vi "Q14070-Z120主界面111.vi"() -> ()   [LabVIEW 2013]
uses:
  <vilib>/printing/EasyPrintingControls.llb/contents.ctl
  <vilib>/printing/EasyPrintingControls.llb/report_type.ctl
  <vilib>/Utility/NIReport.llb/NI_report.lvclass
  <vilib>/printing/EasyPrinting.llb/Easy Print VI Panel or Documentation (path).vi
  PCI8622_32.dll
  <vilib>/Utility/NIReport.llb/NI_ReportGenerationCore.lvlib
panel:
  out "伺服慢进速度":dbl
  out "右伺服慢进位置":dbl format="%#.2f"
  out "左伺服慢进位置":dbl format="%#.2f"
  out "JSSJ":string
  out "FGCS":string
  out "KSSJ":string
  out "本序合格":bool
  out "右压力参数组":dbl[](array[numeric])
  out "右位移参数组":dbl[](array[numeric])
  out "左压力参数组":dbl[](array[numeric])
  out "左位移参数组":dbl[](array[numeric])
  out "右伺服设定走位":dbl
  out "左伺服设定走位":dbl
  out "程序选择-2":bool
  out "程序选择-1":bool
  out "工步提示2":string
  out "工步提示1":string
  in  "报警工步号":u32 caption="工步号1"
  out "报警提示":string
  in  "自动工步号":u32 caption="工步号1"
  out "自动工步提示":string
  in  "产品ID":string="201209190001"
  in  "员工ID":string
  out "员工姓名":string
  in  "电动缸全回零":bool
  in  "电动缸全复位":bool
  out "右伺服快进位置":dbl format="%#.2f"
  out "左伺服快进位置":dbl format="%#.2f"
  out "伺服快进速度":dbl
  out "参数保存错误":errorcluster
  out "传感器保存错误":errorcluster
  out "左实时压力(N)":dbl format="%#.3f"
  out "左实时位移(mm)":dbl=10000.0 format="%#.2f"
  out "右实时位移(mm)":dbl=10000.0 format="%#.2f"
  out "右实时压力(N)":dbl format="%#.3f"
  out "右压装合格":bool
  out "右压装不合格":bool
  out "左压装不合格":bool
  out "左压装合格":bool
  out "监控点最大压力2(KN)":dbl format="%#.3f"
  out "监控点最小压力2(KN)":dbl format="%#.3f"
  out "区域最小压力2(KN)":dbl format="%#.3f"
  out "区域最大压力2(KN)":dbl format="%#.3f"
  out "区域最小位移2(mm)":dbl format="%#.1f"
  out "区域最大位移2(mm)":dbl format="%#.1f"
  out "区域最小压力1(KN)":dbl format="%#.3f"
  out "监控点最大压力1(KN)":dbl format="%#.3f"
  out "监控点最小压力1(KN)":dbl format="%#.3f"
  out "区域最大压力1(KN)":dbl format="%#.3f"
  out "区域最小位移1(mm)":dbl format="%#.1f"
  out "区域最大位移1(mm)":dbl format="%#.1f"
  in  "左工步号2900":u32 caption="工步号1"
  in  "右工步号2700":u32 caption="工步号"
  in  "报警清除":bool
  in  "参数加载":bool
  in  "型号选择":u32(ring) items=["J706", "J709"]
  out "参数加载错误":errorcluster
  in  "停止":bool
  out "ADODB._Connection Out":refnum<k7>
  out "参数查询错误":errorcluster
  in  "联线按钮":bool
  out "通讯状态":bool
  in  "选项卡控件":T1(tab)
  out "左压力位移曲线":cluster{"Y":dbl[], "Y":dbl[]}[](graph) caption="XY图"
  out "右压力位移曲线":cluster{"Y":dbl[], "Y":dbl[]}[](graph) caption="XY图"
  out "压力报警1":bool
  out "压力报警2":bool
  out "左实测监控点压力1(KN)":dbl format="%#.3f"
  out "左实测压入位移(mm)":dbl format="%#.1f"
  out "左实测监控点压力2(KN)":dbl format="%#.3f"
  out "右实测监控点压力2(KN)":dbl format="%#.3f"
  out "右实测压入位移(mm)":dbl format="%#.1f"
  out "右实测监控点压力1(KN)":dbl format="%#.3f"
  out "位移监控点1(mm)":dbl format="%#.2f"
  out "位移监控点2(mm)":dbl format="%#.2f"
  out "右电动缸零位":bool
  out "左电动缸下限":bool
  out "右气缸下降":bool
  out "右气缸上升":bool
  out "右气缸下位":bool
  out "右气缸上位":bool
  out "左气缸上升":bool
  out "左气缸下降":bool
  out "左气缸上位":bool
  out "左气缸下位":bool
  out "左电动缸零位":bool
  out "右电动缸上限":bool
  out "右电动缸下限":bool
  out "左电动缸上限":bool
  in  "顶升气缸上升-右":bool
  in  "顶升气缸下降-右":bool
  in  "顶升气缸上升-左":bool
  in  "顶升气缸下降-左":bool
  out "启动2按钮":bool
  out "启动1按钮":bool
  out "手动/自动":bool
  out "复位按钮":bool
  in  "电动缸下降-右":bool
  in  "电动缸上升-右":bool
  in  "电动缸下降-左":bool
  in  "电动缸上升-左":bool
  in  "电动缸回零-右":bool
  in  "电动缸回零-左":bool
  in  "电动缸复位-左":bool
  in  "电动缸复位-右":bool
  out "急停按钮":bool
  out "安全光幕":bool
  out "气压报警":bool
  in  "右伺服设定走位":dbl caption="右伺服设定走位负值"
  in  "左伺服设定走位":dbl caption="左伺服设定走位负值"
  in  "电动缸绝对移动调试-右":bool
  in  "电动缸绝对移动调试-左":bool
  out "左伺服实时位置":dbl
  out "右伺服实时位置":dbl
  in  "电动缸复位-右 2":bool
  in  "电动缸复位-左 2":bool
  in  "电动缸回零-左 2":bool
  in  "电动缸回零-右 2":bool
  in  "电动缸下降-右 2":bool
  in  "电动缸上升-右 2":bool
  in  "电动缸下降-左 2":bool
  in  "电动缸上升-左 2":bool
  in  "传感器参数保存":bool
  in  "压力1零点偏移值":dbl format="%#.3f"
  in  "压力1比例偏移值":dbl format="%#.3f"
  in  "左位移比例偏移值":dbl format="%#.3f"
  in  "左位移零点偏移值":dbl format="%#.3f"
  in  "压力2零点偏移值":dbl format="%#.3f"
  in  "压力2比例偏移值":dbl format="%#.3f"
  in  "右位移比例偏移值":dbl format="%#.3f"
  in  "右位移零点偏移值":dbl format="%#.3f"
  in  "参数保存":bool
  in  "参数查询":bool
  in  "参数列表":string[][](table)
  # "Q14070-Z120压减震套"
  # "Copying (C) 2014 湖北唯思凌科装备制造有限公司 版权所有"
  # "此界面供伺服定位用，正常生产时 禁止操作！！！"
  # "传感器校验区"
  # "关于传感器校验：\n1、传感器校验需要由具备资质的单位或部门进行校验。\n2、具备权限的用户才能够修改传感器校验参数和试验参数。\n3、修改校验参数方法：先将比例偏移置为1，修改零点偏移，使零点值与校验的传感器一致；然后根据增幅调整比例偏移。"
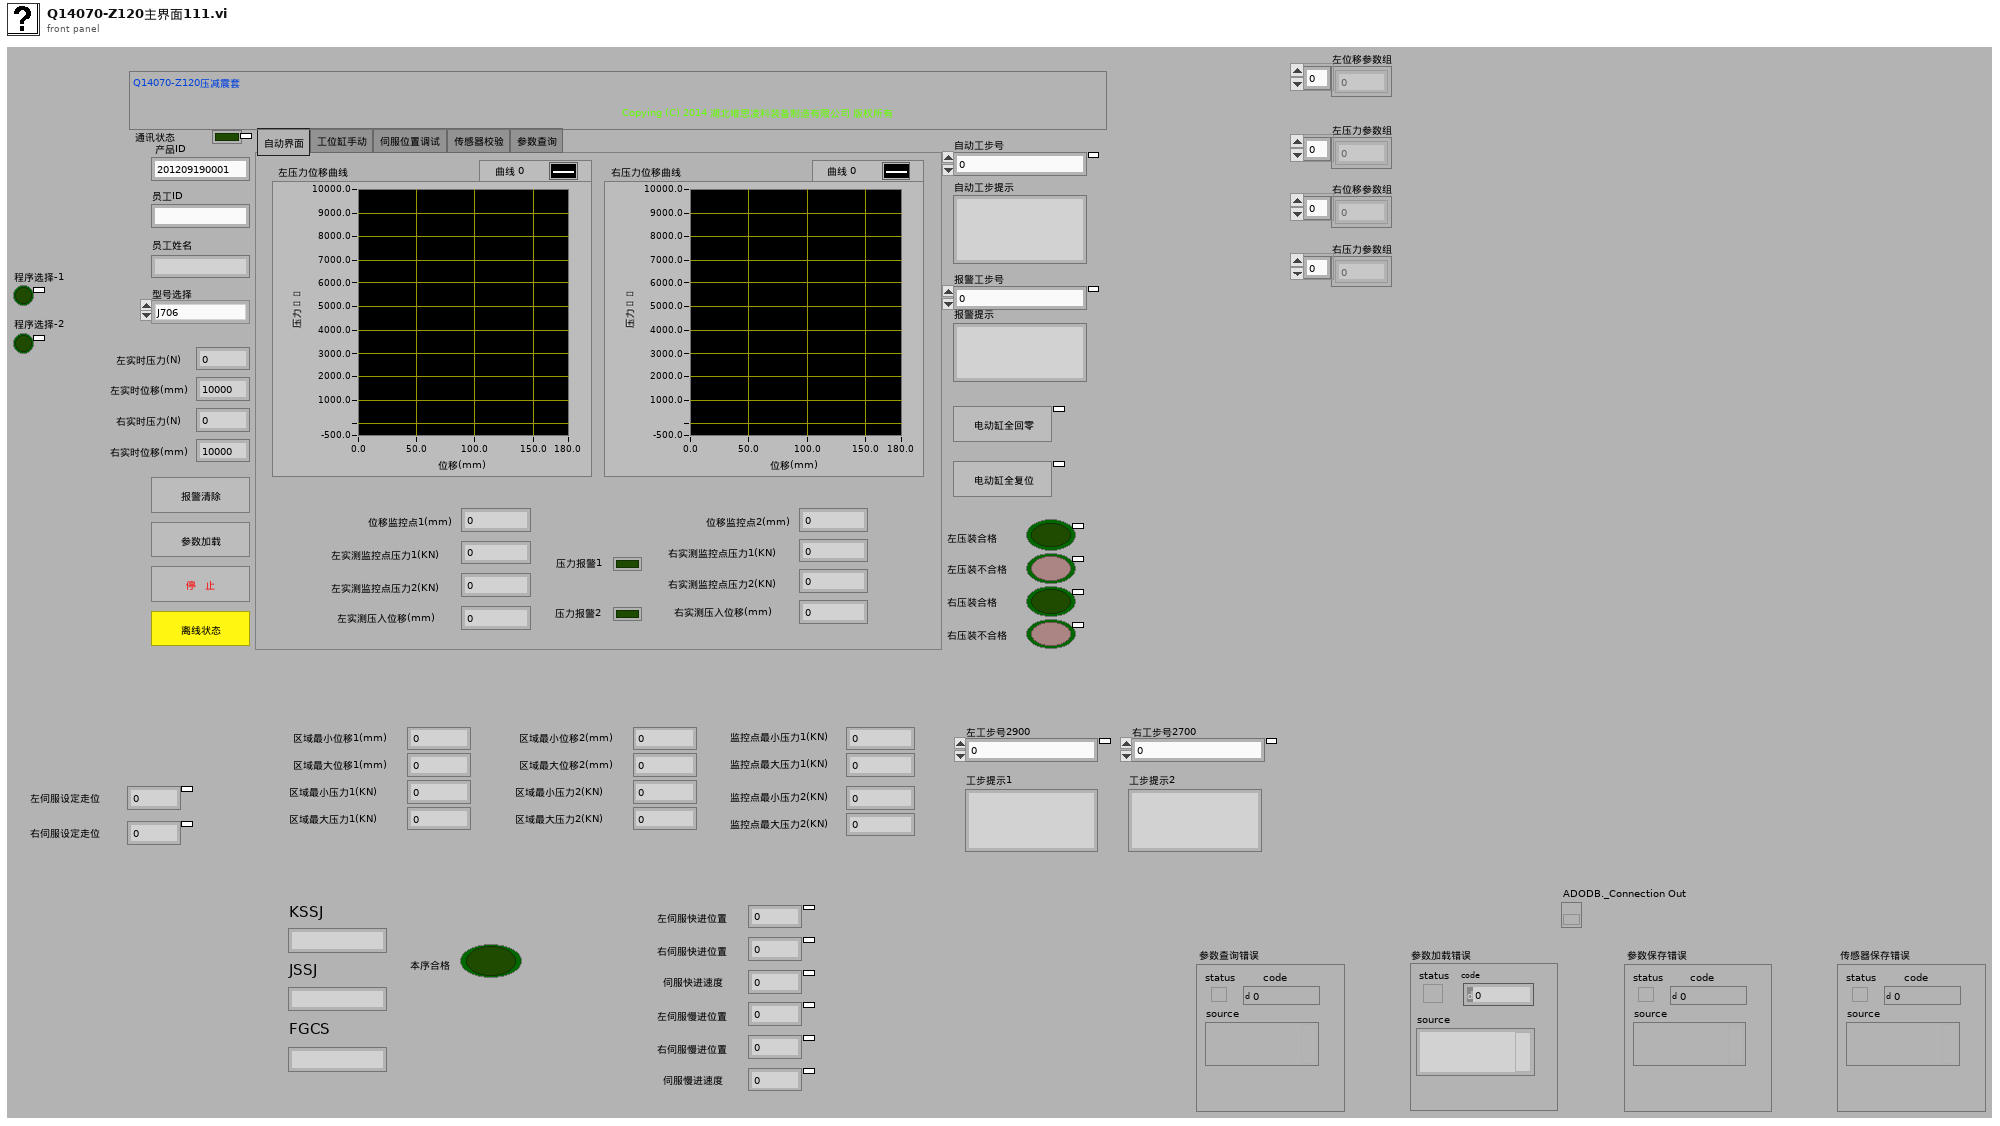
[diagram p1: front panel]
types:
  T1 = enum32{"自动界面", "工位缸手动", "伺服位置调试", "传感器校验", "参数查询"}
  T2 = enum32{"invalid app kind", "Development System", "Run Time System", "Student Edition", "Embedded LabVIEW", "Evaluation", "Custom"}
  T3 = typedef "NI_ReportGenerationCore.lvlib/report_type.ctl" = u16
  T4 = typedef "NI_ReportGenerationCore.lvlib/contents.ctl" = u16
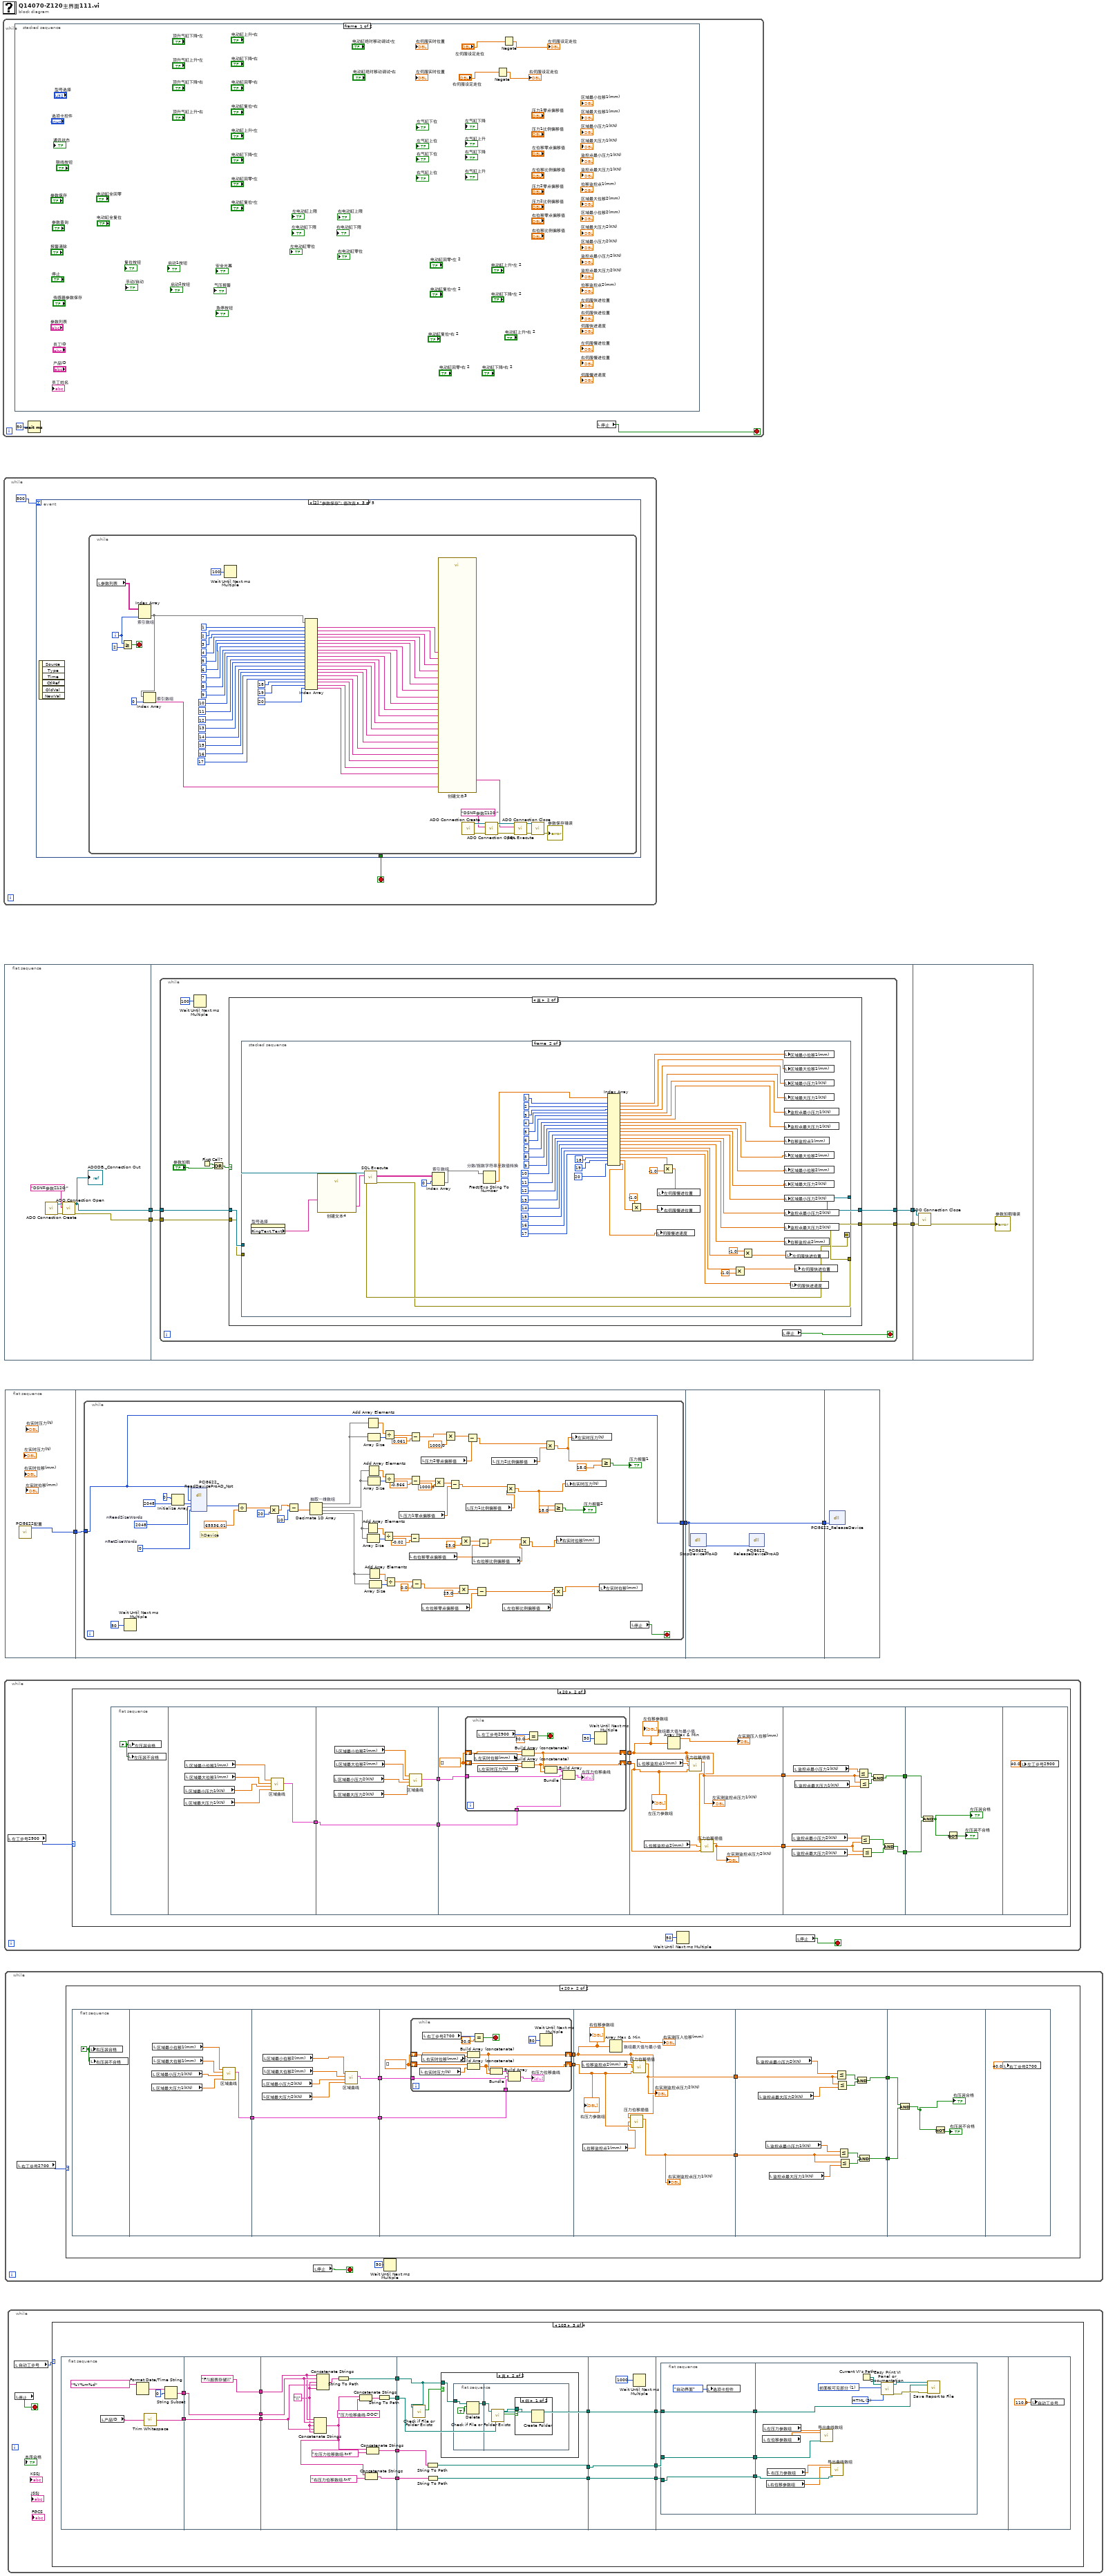
[diagram p0: block diagram]
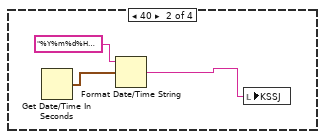
[diagram p3: hidden frame]
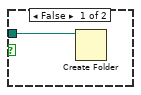
[diagram p4: hidden frame]
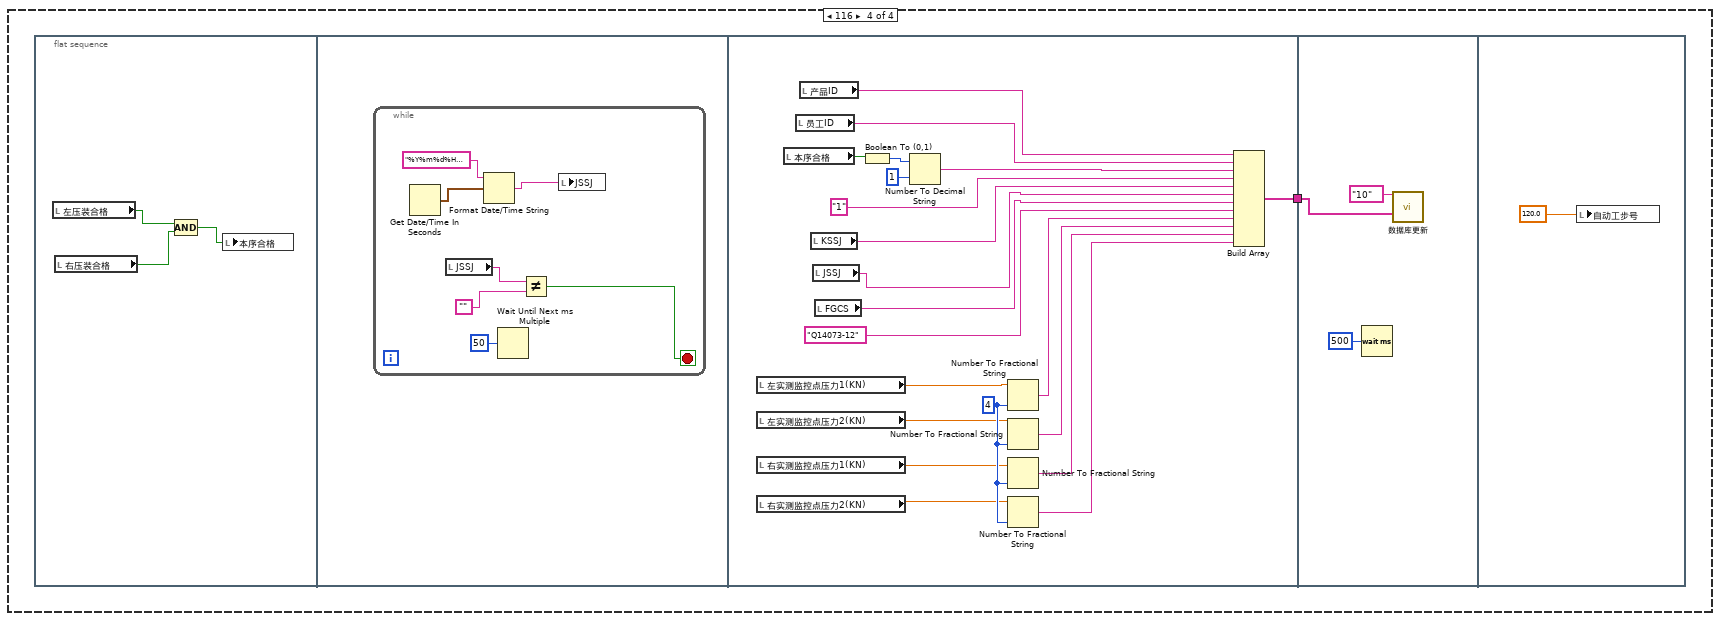
[diagram p6: hidden frame]
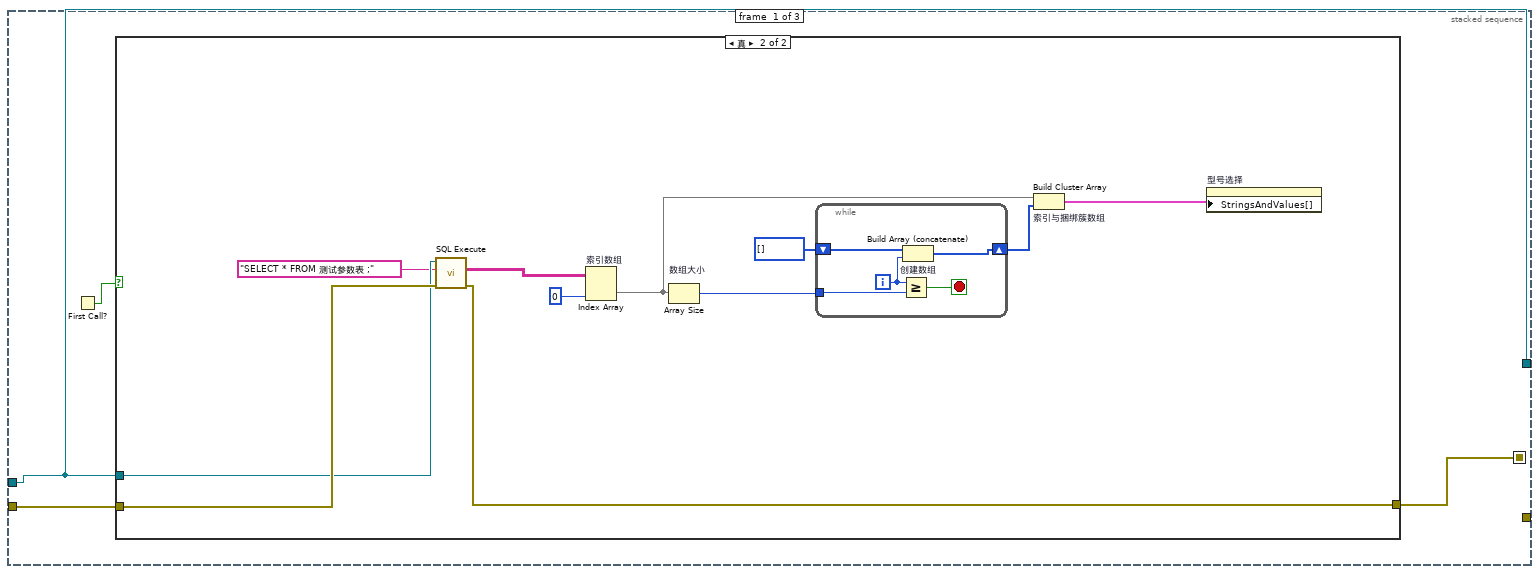
[diagram p10: hidden frame]
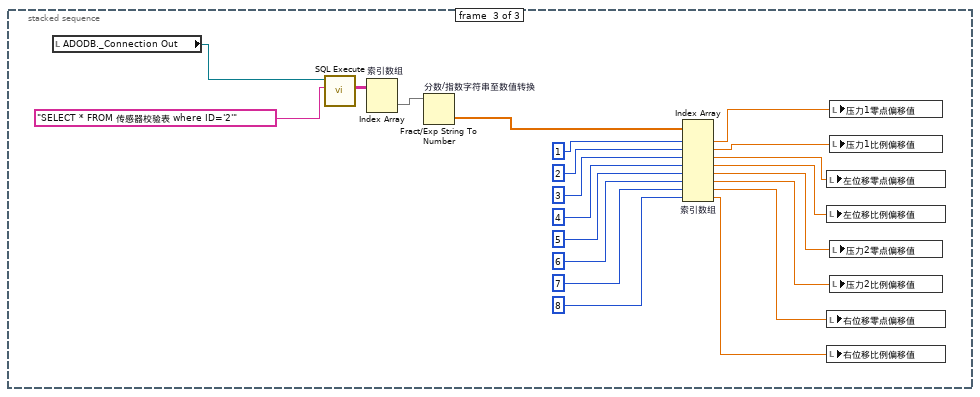
[diagram p12: hidden frame]
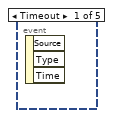
[diagram p13: hidden frame]
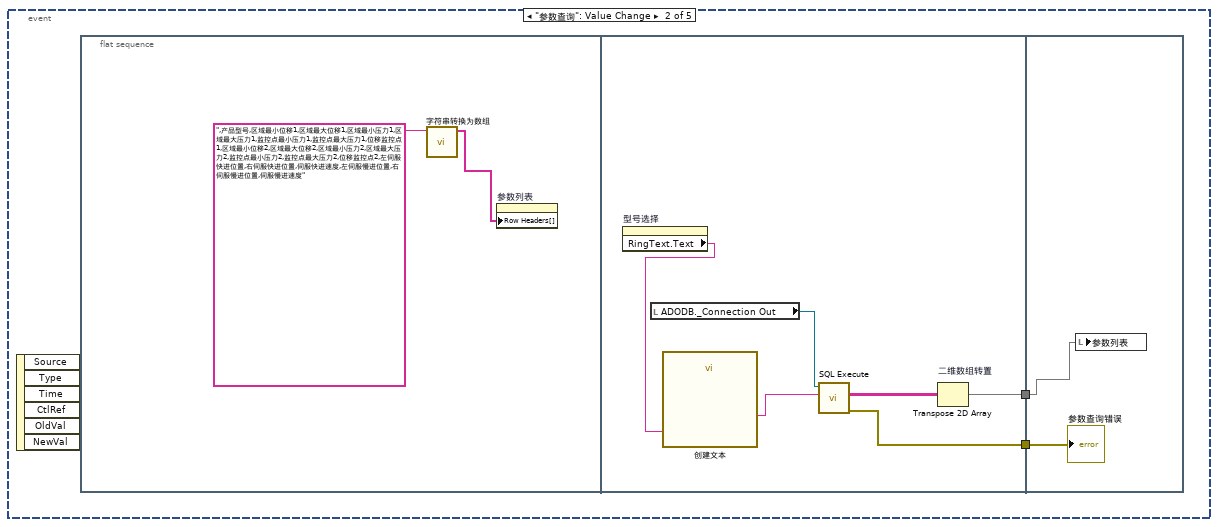
[diagram p14: hidden frame]
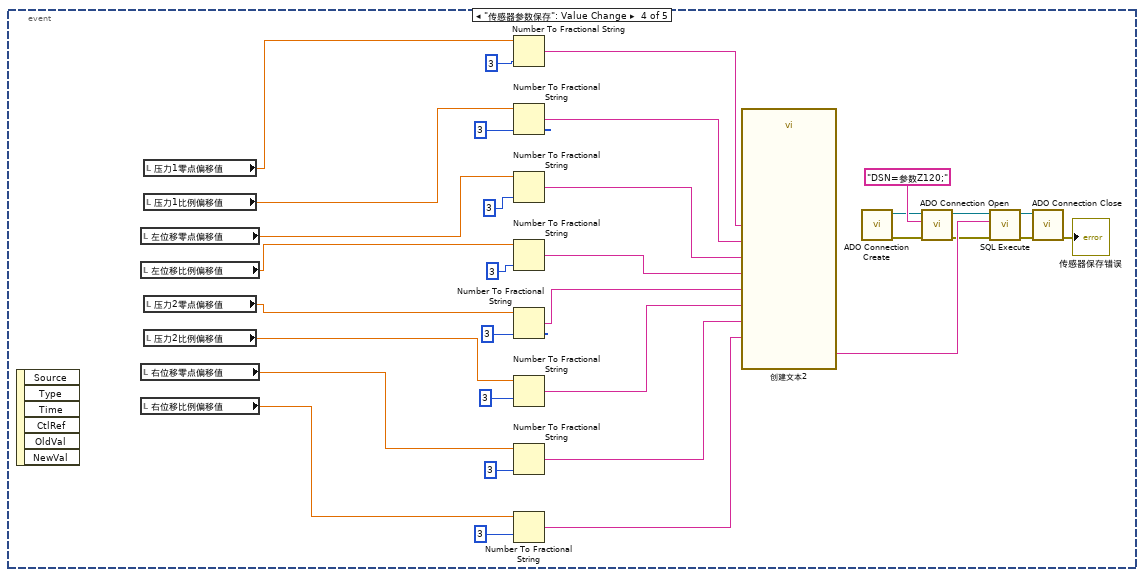
[diagram p15: hidden frame]
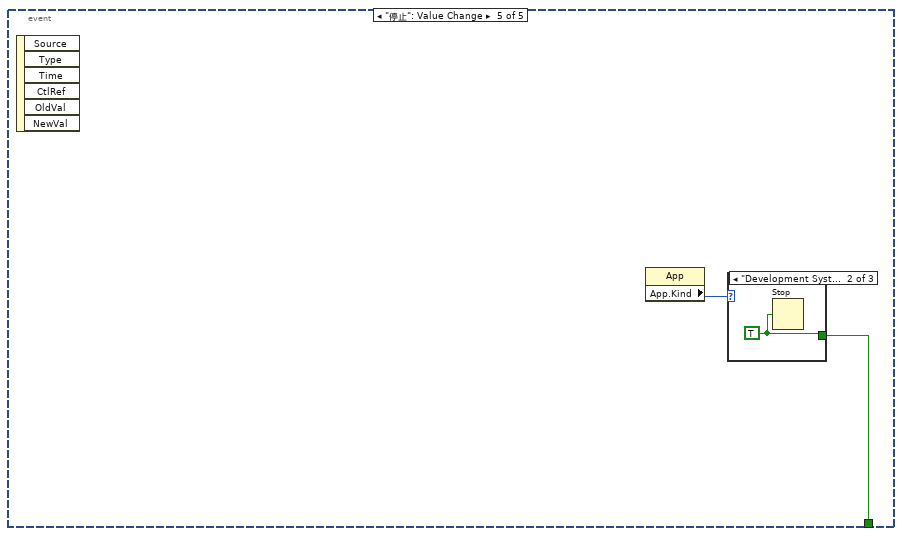
[diagram p16: hidden frame]
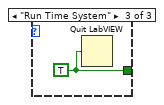
[diagram p18: hidden frame]
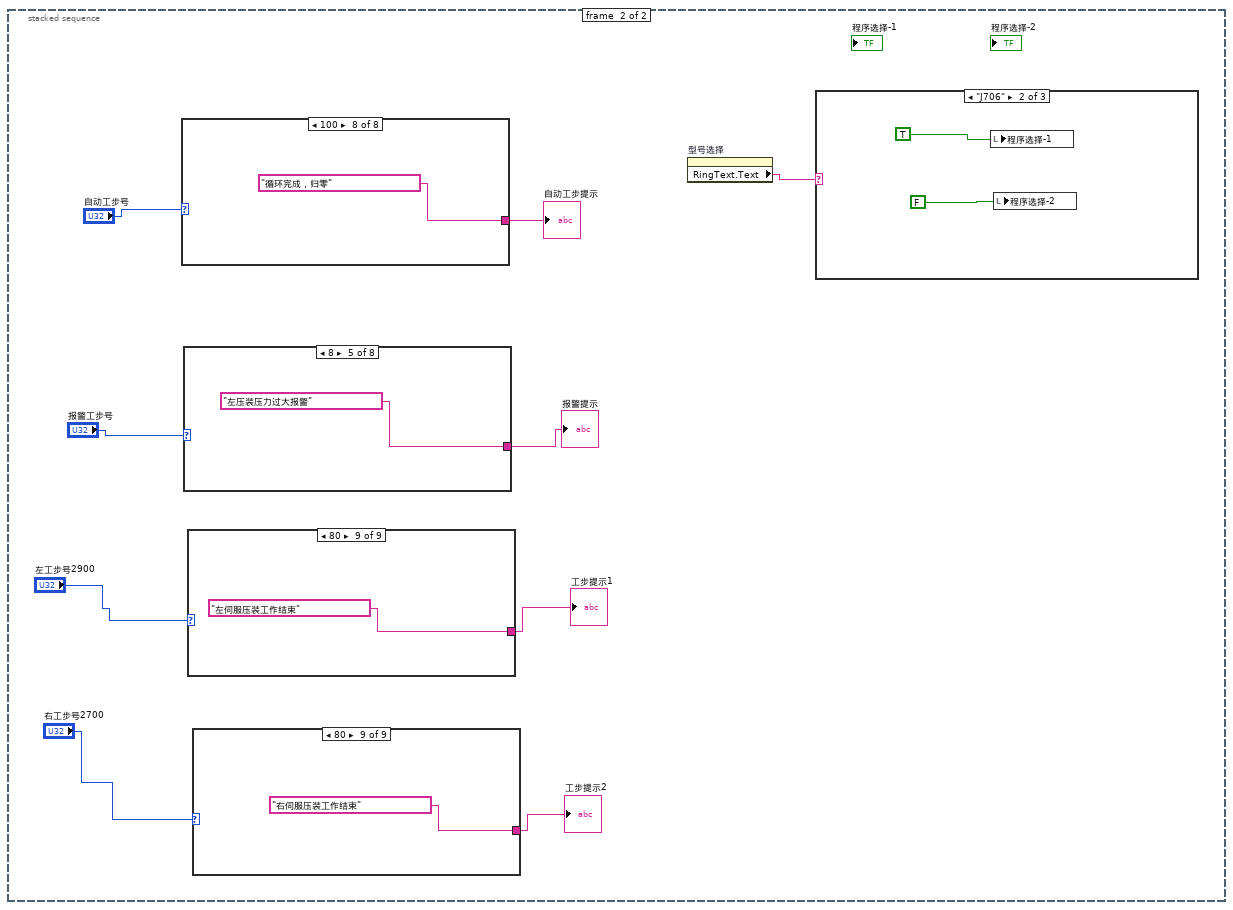
[diagram p19: hidden frame]
diagram:
  n1 = while {
    stop <- w8 stop-if-true
    n2 = stacked-sequence {
      frame #0 {
        n3 = Negate(x="右伺服设定走位") -> (-x=→"右伺服设定走位":dbl)
        n4 = Negate(x="左伺服设定走位") -> (-x=→"左伺服设定走位":dbl)
      }
      frame #1 {
        n5 = case shown="100" "自动工步号" {
          tunnel: ["放入工件，减震套，准备开始" "双手启动开始" "电动缸下降开始" "电动缸下降完成" "电动缸开始回零" "电动缸回零完成，顶升气缸顶升" "顶升气缸下降" "循环完成，归零"] -> w21
          frame 0, Default {
          }
          frame 40 {
          }
          frame 50 {
          }
          frame 60 {
          }
          frame 70 {
          }
          frame 80 {
          }
          frame 90 {
          }
          frame 100 {
          }
        }
        "自动工步提示" <- w21
        n6 = case shown="8" "报警工步号" {
          tunnel: ["工作正常" "压装过程触碰光幕，请急停后复位，并对电动缸回零" "左压装不合格" "右压装不合格" "左压装压力过大报警" "右压装压力过大报警" "左伺服报警，请复位伺服电机" "右伺服报警，请复位伺服电机"] -> w19
          frame 0, Default {
          }
          frame 2 {
          }
          frame 6 {
          }
          frame 7 {
          }
          frame 8 {
          }
          frame 9 {
          }
          frame 11 {
          }
          frame 12 {
          }
        }
        "报警提示" <- w19
        n7 = case shown="80" "左工步号2900" {
          tunnel: ["准备压装" "左伺服压装开始" "左伺服压装中" "左伺服压装结束" "左伺服曲线采集完成" "左伺服回零开始" "左伺服回零中" "左伺服回零完成" "左伺服压装工作结束"] -> w18
          frame 0, Default {
          }
          frame 10 {
          }
          frame 20 {
          }
          frame 30 {
          }
          frame 40 {
          }
          frame 50 {
          }
          frame 60 {
          }
          frame 70 {
          }
          frame 80 {
          }
        }
        "工步提示1" <- w18
        n8 = case shown="80" "右工步号2700" {
          tunnel: ["" "右伺服压装开始" "右伺服压装中" "右伺服压装结束" "右伺服曲线采集完成" "右伺服回零开始" "右伺服回零中" "右伺服回零完成" "右伺服压装工作结束"] -> w17
          frame 0, Default {
          }
          frame 10 {
          }
          frame 20 {
          }
          frame 30 {
          }
          frame 40 {
          }
          frame 50 {
          }
          frame 60 {
          }
          frame 70 {
          }
          frame 80 {
          }
        }
        "工步提示2" <- w17
        n9 = property on="型号选择" class="Ring (严格)"() -> ("RingText.Text"=w14:string)  [unwired: 2 in, 2 out]
        n10 = case shown="\"J706\"" w14 {
          frame "0", Default {
          }
          frame "J706" {
            n11 = local write "程序选择-1"(TRUE ("程序选择-1")) -> ()
            n12 = local write "程序选择-2"(FALSE ("程序选择-2")) -> ()
          }
          frame "J709" {
            n13 = local write "程序选择-1"(FALSE ("程序选择-1")) -> ()
            n14 = local write "程序选择-2"(TRUE ("程序选择-2")) -> ()
          }
        }
      }
    }
    n15 = Wait (ms)(milliseconds to wait=u32 50 ("毫秒倍数")) -> ()  [unwired: 1 out]
    n16 = local read "停止"() -> (w8:bool)
  }
  n17 = while {
    stop <- w61 stop-if-true
    n18 = event shown="[2] \"参数保存\": 值改变" {
      selector: _ -> [_ _ _ _ _]
      dyn-events: _ -> [_ _ _ _ _]
      timeout: 500 -> [_ _ _ _ _]
      tunnel: [_ _ _ _ w165] -> w61
      event Timeout {
        n19 = event-data() -> ()  [unwired: 1 in, 3 out]
      }
      event "参数查询": Value Change {
        n20 = event-data() -> ()  [unwired: 1 in, 6 out]
        n21 = flat-sequence {
          tunnel: [w70] -> w64
          tunnel: [w69] -> w63
          tunnel: w64 -> [w74]
          tunnel: w63 -> [w73]
          frame #0 {
            n22 = call "字符串转换为数组.vi"("查询内容"=",产品型号,区域最小位移1,区域最大位移1,区域最小压力1,区域最大压力1,监控点最小压力1,监控点最大压力1,位移监控点1,区域最小位移2,区域最大位移2,区域最小压力2,区域最大压力2,监控点最小压力2,监控点最大压力2,位移监控点2,左伺服快进位置,右伺服快进位置,伺服快进速度,左伺服慢进位置,右伺服慢进位置,伺服慢进速度") -> ("列首"=w65:string[])  [unwired: 10 in]
            n23 = property on="参数列表" class="Tbl (严格)"("Row Headers[]"=w65) -> ()  [unwired: 2 in, 2 out]
          }
          frame #1 {
            n24 = property on="型号选择" class="Ring (严格)"() -> ("RingText.Text"=w67:string)  [unwired: 2 in, 2 out]
            n25 = local read "ADODB._Connection Out"() -> (w71:refnum<k7>)
            n26 = call "创建文本"("产品型号"=w67) -> ("Result"=w68:string)  [unwired: 13 in, 1 out]
            n27 = call "SQL Execute.vi"("Command Text"=w68, "ADODB._Connection In"=w71) -> ("error out"=w70:errorcluster, "Data"=w72:string[][])  [unwired: 6 in, 2 out]
            n28 = Transpose 2D Array "二维数组转置"(2D array=w72) -> (transposed array=w69:string[][])
          }
          frame #2 {
            n29 = local write "参数列表"(w73) -> ()
            "参数查询错误" <- w74
          }
        }
      }
      event "参数保存": Value Change {
        n30 = event-data() -> ()  [unwired: 1 in, 6 out]
        n31 = while {
          i -> [w126]
          stop <- w128 stop-if-true
          n32 = local read "参数列表"() -> (w82:string[][])
          n33 = Greater Or Equal?(x=w126, y=2) -> (x >= y?=w128:bool)
          n34 = Index Array "索引数组"(array=w82, index (col)=w126) -> (element=w102:string[])  [unwired: 1 in]
          n35 = Index Array "索引数组"(array=w102, index=0 ("索引")) -> (element=w75:string)
          n36 = Wait Until Next ms Multiple(millisecond multiple=u32 100 ("毫秒倍数")) -> ()  [unwired: 1 out]
          n37 = Index Array(array=w102, index #1=1 ("索引"), index #2=2 ("索引"), index #3=3 ("索引"), index #4=4 ("索引"), index #5=5 ("索引"), index #6=6 ("索引"), index #7=7 ("索引"), index #8=8 ("索引"), index #9=9 ("索引"), index #10=10 ("索引"), index #11=11 ("索引"), index #12=12 ("索引"), index #13=13 ("索引"), index #14=14 ("索引"), index #15=15 ("索引"), index #16=16 ("索引"), index #17=17 ("索引"), index #18=18 ("索引"), index #19=19 ("索引"), index #20=20 ("索引")) -> (element #1=w100:string, element #2=w99:string, element #3=w98:string, element #4=w97:string, element #5=w96:string, element #6=w95:string, element #7=w94:string, element #8=w93:string, element #9=w92:string, element #10=w91:string, element #11=w90:string, element #12=w89:string, element #13=w88:string, element #14=w87:string, element #15=w86:string, element #16=w85:string, element #17=w84:string, element #18=w78:string, element #19=w77:string, element #20=w76:string)
          n38 = call "创建文本3"("区域最小位移1"=w100, "区域最大位移1"=w99, "区域最小压力1"=w98, "区域最大压力1"=w97, "监控点最小压力1"=w96, "监控点最大压力1"=w95, "位移监控点1"=w94, "区域最小位移2"=w93, "区域最大位移2"=w92, "区域最小压力2"=w91, "区域最大压力2"=w90, "监控点最小压力2"=w89, "监控点最大压力2"=w88, "位移监控点2"=w87, "左伺服快进位置"=w86, "右伺服快进位置"=w85, "伺服快进速度"=w84, "左伺服慢进位置"=w78, "右伺服慢进位置"=w77, "伺服慢进速度"=w76, "产品型号"=w75) -> ("Result"=w83:string)  [unwired: 5 in, 1 out]
          n39 = call "ADO Connection Create.vi"() -> ("error out"=w122:errorcluster, "ADODB._Connection Out"=w123:refnum<k7>)  [unwired: 10 in]
          n40 = call "ADO Connection Open.vi"("error in (no error)"=w122, "ConnectionString"="DSN=参数Z120;", "ADODB._Connection In"=w123) -> ("error out"=w119:errorcluster, "ADODB._Connection Out"=w120:refnum<k7>)  [unwired: 7 in]
          n41 = call "SQL Execute.vi"("error in (no error)"=w119, "Command Text"=w83, "ADODB._Connection In"=w120) -> ("error out"=w129:errorcluster, "ADODB._Connection Out"=w130:refnum<k7>)  [unwired: 5 in, 2 out]
          n42 = call "ADO Connection Close.vi"("error in (no error)"=w129, "ADODB._Connection In"=w130) -> ("error out"=→"参数保存错误":errorcluster)  [unwired: 8 in, 1 out]
        }
      }
      event "传感器参数保存": Value Change {
        n43 = event-data() -> ()  [unwired: 1 in, 6 out]
        n44 = local read "左位移零点偏移值"() -> (w157:dbl)
        n45 = local read "左位移比例偏移值"() -> (w158:dbl)
        n46 = local read "右位移零点偏移值"() -> (w161:dbl)
        n47 = local read "右位移比例偏移值"() -> (w162:dbl)
        n48 = local read "压力1零点偏移值"() -> (w155:dbl)
        n49 = local read "压力1比例偏移值"() -> (w156:dbl)
        n50 = local read "压力2零点偏移值"() -> (w159:dbl)
        n51 = local read "压力2比例偏移值"() -> (w160:dbl)
        n52 = Number To Fractional String(number=w155, precision (6)=i16 3 ("精度(6)")) -> (F-format string=w147:string)  [unwired: 2 in]
        n53 = Number To Fractional String(number=w156, precision (6)=i16 3 ("精度(6)")) -> (F-format string=w148:string)  [unwired: 2 in]
        n54 = Number To Fractional String(number=w157, precision (6)=i16 3 ("精度(6)")) -> (F-format string=w149:string)  [unwired: 2 in]
        n55 = Number To Fractional String(number=w158, precision (6)=i16 3 ("精度(6)")) -> (F-format string=w150:string)  [unwired: 2 in]
        n56 = Number To Fractional String(number=w159, precision (6)=i16 3 ("精度(6)")) -> (F-format string=w151:string)  [unwired: 2 in]
        n57 = Number To Fractional String(number=w160, precision (6)=i16 3 ("精度(6)")) -> (F-format string=w152:string)  [unwired: 2 in]
        n58 = Number To Fractional String(number=w161, precision (6)=i16 3 ("精度(6)")) -> (F-format string=w153:string)  [unwired: 2 in]
        n59 = Number To Fractional String(number=w162, precision (6)=i16 3 ("精度(6)")) -> (F-format string=w154:string)  [unwired: 2 in]
        n60 = call "创建文本2"("左位移比例偏移值"=w150, "压力2比例偏移值"=w152, "右位移比例偏移值"=w154, "压力1零点偏移值"=w147, "压力1比例偏移值"=w148, "左位移零点偏移值"=w149, "压力2零点偏移值"=w151, "右位移零点偏移值"=w153) -> ("Result"=w163:string)  [unwired: 6 in, 1 out]
        n61 = call "ADO Connection Create.vi"() -> ("error out"=w136:errorcluster, "ADODB._Connection Out"=w134:refnum<k7>)  [unwired: 10 in]
        n62 = call "ADO Connection Open.vi"("error in (no error)"=w136, "ConnectionString"="DSN=参数Z120;", "ADODB._Connection In"=w134) -> ("error out"=w137:errorcluster, "ADODB._Connection Out"=w135:refnum<k7>)  [unwired: 7 in]
        n63 = call "SQL Execute.vi"("error in (no error)"=w137, "Command Text"=w163, "ADODB._Connection In"=w135) -> ("error out"=w133:errorcluster, "ADODB._Connection Out"=w132:refnum<k7>)  [unwired: 5 in, 2 out]
        n64 = call "ADO Connection Close.vi"("error in (no error)"=w133, "ADODB._Connection In"=w132) -> ("error out"=→"传感器保存错误":errorcluster)  [unwired: 8 in, 1 out]
      }
      event "停止": Value Change {
        n65 = event-data() -> ()  [unwired: 1 in, 6 out]
        n66 = property on="属性节点" class="App"() -> ("App.Kind"=w166:T2)  [unwired: 2 in, 2 out]
        n67 = case shown="\"Development System\"" w166 {
          tunnel: [_ w167 w168] -> w165
          frame "invalid app kind", Default {
          }
          frame "Development System" {
            w167 = TRUE ("停止？(T)")
            n68 = Stop(stop? (T)=w167) -> ()
          }
          frame "Run Time System" {
            w168 = TRUE ("退出？(T)")
            n69 = Quit LabVIEW(quit? (T)=w168) -> ()
          }
        }
      }
    }
  }
  n70 = while {
    stop <- w171 stop-if-true
    n71 = local read "左工步号2900"() -> (w169:u32)
    n72 = case shown="20" w169 {
      frame 0, Default {
      }
      frame 20 {
        n73 = flat-sequence {
          tunnel: [w186] -> w176
          tunnel: w176 -> [w192]
          tunnel: [w192] -> w175
          tunnel: [w187] -> w174
          tunnel: [w196] -> w180
          tunnel: [w195] -> w179
          tunnel: w175 -> [w194]
          tunnel: w174 -> [w193]
          tunnel: w180 -> [w214]
          tunnel: w179 -> [w213]
          tunnel: [w217] -> w178
          tunnel: [w212] -> w172
          tunnel: w178 -> [w230]
          tunnel: [w225] -> w177
          tunnel: [w222] -> w173
          tunnel: w172 -> [w219]
          tunnel: w177 -> [w233]
          tunnel: w173 -> [w232]
          frame #0 {
            w181 = FALSE ("压装合格1")
            n74 = local write "左压装不合格"(w181) -> ()
            n75 = local write "左压装合格"(w181) -> ()
          }
          frame #1 {
            n76 = local read "区域最小压力1(KN)"() -> (w183:dbl)
            n77 = local read "区域最大压力1(KN)"() -> (w182:dbl)
            n78 = local read "区域最小位移1(mm)"() -> (w185:dbl)
            n79 = local read "区域最大位移1(mm)"() -> (w184:dbl)
            n80 = call "区域曲线.vi"("区域最大压力(N)"=w182, "区域最小压力(N)"=w183, "区域最大位移(mm)"=w184, "区域最小位移(mm)"=w185) -> ("区域曲线"=w186:cluster{dbl[], dbl[]})  [unwired: 7 in]
          }
          frame #2 {
            n81 = local read "区域最小压力2(KN)"() -> (w189:dbl)
            n82 = local read "区域最大压力2(KN)"() -> (w188:dbl)
            n83 = local read "区域最小位移2(mm)"() -> (w191:dbl)
            n84 = local read "区域最大位移2(mm)"() -> (w190:dbl)
            n85 = call "区域曲线.vi"("区域最大压力(N)"=w188, "区域最小压力(N)"=w189, "区域最大位移(mm)"=w190, "区域最小位移(mm)"=w191) -> ("区域曲线"=w187:cluster{dbl[], dbl[]})  [unwired: 7 in]
          }
          frame #3 {
            w197 = dbl[] []
            n86 = while {
              shift-right: [w209] -> w196
              shift-left: w197 -> [w210]
              shift-right: [w207] -> w195
              shift-left: w197 -> [w208]
              tunnel: w194 -> [w198]
              tunnel: w193 -> [w199]
              stop <- w202 stop-if-true
              n87 = local read "左实时位移(mm)"() -> (w206:dbl)
              n88 = local read "左工步号2900"() -> (w204:u32)
              n89 = local read "左实时压力(N)"() -> (w205:dbl)
              n90 = Build Array (concatenate)(w210, w206) -> (w209:dbl[])
              n91 = Build Array (concatenate)(w208, w205) -> (w207:dbl[])
              n92 = Equal?(x=w204, y=30.0) -> (x = y?=w202:bool)
              n93 = Bundle(w209, w207) -> (w211:cluster{dbl[], dbl[]})  [unwired: 1 in]
              n94 = Build Array(w211, w199, w198) -> (→"左压力位移曲线":cluster{dbl[], dbl[]}[])
              n95 = Wait Until Next ms Multiple(millisecond multiple=u32 50 ("毫秒倍数")) -> ()  [unwired: 1 out]
            }
          }
          frame #4 {
            n96 = local read "位移监控点1(mm)"() -> (w218:dbl)
            n97 = local read "位移监控点2(mm)"() -> (w215:dbl)
            n98 = Array Max & Min "数组最大值与最小值"(array=w214) -> (max value=→"左实测压入位移(mm)":dbl)  [unwired: 3 out]
            n99 = call "压力位移插值.vi"("压力数组"=w213, "监控点位移"=w218, "位移数组"=w214) -> ("监控点压力"=w217:dbl)  [unwired: 2 in]
            "左实测监控点压力1(KN)" <- w217
            n100 = call "压力位移插值.vi"("压力数组"=w213, "监控点位移"=w215, "位移数组"=w214) -> ("监控点压力"=w212:dbl)  [unwired: 2 in]
            "左实测监控点压力2(KN)" <- w212
            "左位移参数组" <- w214
            "左压力参数组" <- w213
          }
          frame #5 {
            n101 = local read "监控点最小压力2(KN)"() -> (w227:dbl)
            n102 = local read "监控点最大压力2(KN)"() -> (w226:dbl)
            n103 = local read "监控点最小压力1(KN)"() -> (w229:dbl)
            n104 = local read "监控点最大压力1(KN)"() -> (w228:dbl)
            n105 = Less Or Equal?(x=w229, y=w230) -> (x <= y?=w224:bool)
            n106 = Less Or Equal?(x=w230, y=w228) -> (x <= y?=w223:bool)
            n107 = Less Or Equal?(x=w227, y=w219) -> (x <= y?=w221:bool)
            n108 = Less Or Equal?(x=w219, y=w226) -> (x <= y?=w220:bool)
            n109 = And(x=w224, y=w223) -> (x .and. y?=w225:bool)
            n110 = And(x=w221, y=w220) -> (x .and. y?=w222:bool)
          }
          frame #6 {
            n111 = And(x=w233, y=w232) -> (x .and. y?=w231:bool)
            "左压装合格" <- w231
            n112 = Not(x=w231) -> (.not. x?=→"左压装不合格":bool)
          }
          frame #7 {
            n113 = local write "左工步号2900"(40.0 ("工步2序号")) -> ()
          }
        }
      }
    }
    n114 = Wait Until Next ms Multiple(millisecond multiple=u32 50 ("毫秒倍数")) -> ()  [unwired: 1 out]
    n115 = local read "停止"() -> (w171:bool)
  }
  n116 = flat-sequence {
    tunnel: [w236] -> w7
    tunnel: [w237] -> w6
    tunnel: w7 -> [w244]
    tunnel: w6 -> [w243]
    tunnel: [w242] -> w5
    tunnel: [w241] -> w4
    tunnel: w5 -> [w360]
    tunnel: w4 -> [w359]
    frame #0 {
      n117 = call "ADO Connection Create.vi"() -> ("error out"=w239:errorcluster, "ADODB._Connection Out"=w240:refnum<k7>)  [unwired: 10 in]
      n118 = call "ADO Connection Open.vi"("error in (no error)"=w239, "ConnectionString"="DSN=参数Z120;", "ADODB._Connection In"=w240) -> ("error out"=w237:errorcluster, "ADODB._Connection Out"=w236:refnum<k7>)  [unwired: 7 in]
      "ADODB._Connection Out" <- w236
    }
    frame #1 {
      n119 = while {
        tunnel: w244 -> [w253]
        tunnel: w243 -> [w252]
        tunnel: [w251] -> w242
        tunnel: [w250] -> w241
        stop <- w246 stop-if-true
        n120 = Wait Until Next ms Multiple(millisecond multiple=u32 100 ("毫秒倍数")) -> ()  [unwired: 1 out]
        n121 = First Call?() -> (First Call?: T/F=w249:bool)
        n122 = Or(x=w249, y="参数加载") -> (x .or. y?=w248:bool)
        n123 = case shown="真" w248 {
          tunnel: w253 -> [w255 w259]
          tunnel: w252 -> [w254 w258]
          tunnel: [w255 w257] -> w251
          tunnel: [w254 w256] -> w250
          frame False {
          }
          frame True {
            n124 = stacked-sequence {
              seq-local: [w261 _ _] -> [_ w335 _]
              tunnel: w259 -> [w262 w332 _]
              tunnel: w258 -> [w263 _ _]
              tunnel: [w262 _ _] -> w257
              tunnel: [_ w334 _] -> w256
              frame #0 {
                n125 = First Call?() -> (First Call?: T/F=w260:bool)
                n126 = case shown="真" w260 {
                  tunnel: w263 -> [w264 w275]
                  tunnel: w262 -> [_ w274]
                  tunnel: [w264 w273] -> w261
                  frame False {
                  }
                  frame True {
                    n127 = call "SQL Execute.vi"("error in (no error)"=w275, "Command Text"="SELECT * FROM 测试参数表 ;", "ADODB._Connection In"=w274) -> ("error out"=w273:errorcluster, "Data"=w267:string[][])  [unwired: 5 in, 2 out]
                    n128 = Index Array "索引数组"(array=w267, index (col)=0 ("禁用的索引 (列)")) -> (element=w270:string[])  [unwired: 1 in]
                    n129 = Array Size "数组大小"(array=w270) -> (size(s)=w269:i32)
                    n130 = while {
                      shift-right: [w278] -> w268
                      shift-left: i32[] [] -> [w279]
                      tunnel: w269 -> [w276]
                      i -> [w277]
                      stop <- w280 stop-if-true
                      n131 = Greater Or Equal?(x=w277, y=w276) -> (x >= y?=w280:bool)
                      n132 = Build Array (concatenate) "创建数组"(w279, w277) -> (w278:i32[])
                    }
                    n133 = Build Cluster Array "索引与捆绑簇数组"(w270, w268) -> (w265:cluster{"String":string, i32}[])
                    n134 = property on="型号选择" class="Ring (严格)"("StringsAndValues[]"=w265) -> ()  [unwired: 2 in, 2 out]
                  }
                }
              }
              frame #1 {
                n135 = property on="型号选择" class="Ring (严格)"() -> ("RingText.Text"=w330:string)  [unwired: 2 in, 2 out]
                n136 = call "创建文本4"("产品型号"=w330) -> ("Result"=w333:string)  [unwired: 13 in, 1 out]
                n137 = call "SQL Execute.vi"("error in (no error)"=w335, "Command Text"=w333, "ADODB._Connection In"=w332) -> ("error out"=w334:errorcluster, "Data"=w337:string[][])  [unwired: 5 in, 2 out]
                n138 = Index Array "索引数组"(array=w337, index (row)=0 ("索引 (行)")) -> (element=w331:string[])  [unwired: 1 in]
                n139 = Fract/Exp String To Number "分数/指数字符串至数值转换"(string=w331) -> (number=w312:dbl[])  [unwired: 3 in, 1 out]
                n140 = Index Array(array=w312, index #1=1 ("索引"), index #2=2 ("索引"), index #3=3 ("索引"), index #4=4 ("索引"), index #5=5 ("索引"), index #6=6 ("索引"), index #7=7 ("索引"), index #8=8 ("索引"), index #9=9 ("索引"), index #10=10 ("索引"), index #11=11 ("索引"), index #12=12 ("索引"), index #13=13 ("索引"), index #14=14 ("索引"), index #15=15 ("索引"), index #16=16 ("索引"), index #17=17 ("索引"), index #18=18 ("索引"), index #19=19 ("索引"), index #20=20 ("索引")) -> (element #1=w311:dbl, element #2=w310:dbl, element #3=w309:dbl, element #4=w308:dbl, element #5=w307:dbl, element #6=w306:dbl, element #7=w305:dbl, element #8=w304:dbl, element #9=w303:dbl, element #10=w302:dbl, element #11=w301:dbl, element #12=w300:dbl, element #13=w299:dbl, element #14=w298:dbl, element #15=w297:dbl, element #16=w296:dbl, element #17=w295:dbl, element #18=w287:dbl, element #19=w286:dbl, element #20=w285:dbl)
                n141 = Multiply(x=-1.0, y=w286) -> (x*y=w282:dbl)
                n142 = local write "伺服慢进速度"(w285) -> ()
                n143 = local write "右伺服慢进位置"(w282) -> ()
                n144 = Multiply(x=w287, y=-1.0) -> (x*y=w284:dbl)
                n145 = local write "左伺服慢进位置"(w284) -> ()
                n146 = Multiply(x=w296, y=-1.0) -> (x*y=w292:dbl)
                n147 = Multiply(x=-1.0, y=w297) -> (x*y=w294:dbl)
                n148 = local write "区域最小位移1(mm)"(w311) -> ()
                n149 = local write "区域最大位移1(mm)"(w310) -> ()
                n150 = local write "区域最小压力1(KN)"(w309) -> ()
                n151 = local write "区域最大压力1(KN)"(w308) -> ()
                n152 = local write "监控点最小压力1(KN)"(w307) -> ()
                n153 = local write "监控点最大压力1(KN)"(w306) -> ()
                n154 = local write "位移监控点1(mm)"(w305) -> ()
                n155 = local write "区域最大位移2(mm)"(w304) -> ()
                n156 = local write "区域最小位移2(mm)"(w303) -> ()
                n157 = local write "区域最大压力2(KN)"(w302) -> ()
                n158 = local write "区域最小压力2(KN)"(w301) -> ()
                n159 = local write "监控点最小压力2(KN)"(w300) -> ()
                n160 = local write "监控点最大压力2(KN)"(w299) -> ()
                n161 = local write "位移监控点2(mm)"(w298) -> ()
                n162 = local write "左伺服快进位置"(w294) -> ()
                n163 = local write "伺服快进速度"(w295) -> ()
                n164 = local write "右伺服快进位置"(w292) -> ()
              }
              frame #2 {
                n165 = local read "ADODB._Connection Out"() -> (w350:refnum<k7>)
                n166 = call "SQL Execute.vi"("Command Text"="SELECT * FROM 传感器校验表 where ID='2'", "ADODB._Connection In"=w350) -> ("Data"=w351:string[][])  [unwired: 6 in, 3 out]
                n167 = Index Array "索引数组"(array=w351) -> (element=w352:string[])  [unwired: 2 in]
                n168 = Fract/Exp String To Number "分数/指数字符串至数值转换"(string=w352) -> (number=w353:dbl[])  [unwired: 3 in, 1 out]
                n169 = Index Array "索引数组"(array=w353, index #1=1 ("索引"), index #2=2 ("索引"), index #3=3 ("索引"), index #4=4 ("索引"), index #5=5 ("索引"), index #6=6 ("索引"), index #7=7 ("索引"), index #8=8 ("索引")) -> (element #1=w345:dbl, element #2=w344:dbl, element #3=w343:dbl, element #4=w342:dbl, element #5=w341:dbl, element #6=w340:dbl, element #7=w339:dbl, element #8=w338:dbl)
                n170 = local write "左位移零点偏移值"(w343) -> ()
                n171 = local write "左位移比例偏移值"(w342) -> ()
                n172 = local write "右位移零点偏移值"(w339) -> ()
                n173 = local write "右位移比例偏移值"(w338) -> ()
                n174 = local write "压力1零点偏移值"(w345) -> ()
                n175 = local write "压力1比例偏移值"(w344) -> ()
                n176 = local write "压力2零点偏移值"(w341) -> ()
                n177 = local write "压力2比例偏移值"(w340) -> ()
              }
            }
          }
        }
        n178 = local read "停止"() -> (w246:bool)
      }
    }
    frame #2 {
      n179 = call "ADO Connection Close.vi"("error in (no error)"=w359, "ADODB._Connection In"=w360) -> ("error out"=→"参数加载错误":errorcluster)  [unwired: 8 in, 1 out]
    }
  }
  n180 = flat-sequence {
    tunnel: [w362] -> w3
    tunnel: w3 -> [w364]
    tunnel: [w363] -> w2
    tunnel: w2 -> [w432]
    tunnel: [w432] -> w1
    tunnel: w1 -> [w434]
    frame #0 {
      n181 = call "PCI8622配置.vi"() -> ("DeviceID"=w362:i32)  [unwired: 11 in]
    }
    frame #1 {
      n182 = while {
        tunnel: w364 -> [w391]
        tunnel: [w391] -> w363
        stop <- w382 stop-if-true
        w430 = 0  # nRetSizeWords
        w431 = 2048  # nReadSizeWords
        # "hDevice"
        n183 = Wait Until Next ms Multiple(millisecond multiple=u32 50 ("毫秒倍数")) -> ()  [unwired: 1 out]
        n184 = Initialize Array(u16 0, 2048 ("dimension size")) -> (w423:u16[])
        n185 = dll-call lib="PTH17abs DQ14070-Z120人机界面-Z120PCI8622_32.dll" fn="PCI8622_ReadDeviceProAD_Npt" label="ReadDeviceProAD_Npt"("hDevice"=w391, "ADBuffer[]"=w423, "nReadSizeWords"=w431, "nRetSizeWords"=w430) -> ("ADBuffer[]"=w426:u16[])  [unwired: 7 in, 2 out]
        n186 = Divide(x=w426, y=65536.01) -> (x/y=w427:dbl[])
        n187 = Multiply(x=w427, y=20) -> (x*y=w368:dbl[])
        n188 = Subtract(x=w368, y=10) -> (x-y=w369:dbl[])
        n189 = Decimate 1D Array "抽取一维数组"(w369) -> (w419:dbl[], w406:dbl[], w396:dbl[], w395:dbl[])
        n190 = Add Array Elements(numeric array=w396) -> (sum=w393:dbl)
        n191 = Add Array Elements(numeric array=w419) -> (sum=w420:dbl)
        n192 = Array Size(array=w396) -> (size(s)=w405:i32)
        n193 = Add Array Elements(numeric array=w406) -> (sum=w412:dbl)
        n194 = Array Size(array=w419) -> (size(s)=w421:i32)
        n195 = Array Size(array=w406) -> (size(s)=w413:i32)
        n196 = Add Array Elements(numeric array=w395) -> (sum=w392:dbl)
        n197 = Array Size(array=w395) -> (size(s)=w394:i32)
        n198 = Divide(x=w393, y=w405) -> (x/y=w404:dbl)
        n199 = Divide(x=w420, y=w421) -> (x/y=w417:dbl)
        n200 = Divide(x=w412, y=w413) -> (x/y=w410:dbl)
        n201 = Divide(x=w392, y=w394) -> (x/y=w400:dbl)
        n202 = local read "压力1零点偏移值"() -> (w376:dbl)
        n203 = Subtract(x=w404, y=-0.02) -> (x-y=w386:dbl)
        n204 = local read "右位移零点偏移值"() -> (w373:dbl)
        n205 = Subtract(x=w417, y=0.061) -> (x-y=w415:dbl)
        n206 = Subtract(x=w410, y=-0.566) -> (x-y=w408:dbl)
        n207 = Subtract(x=w400, y=0.0) -> (x-y=w384:dbl)
        n208 = local read "压力2零点偏移值"() -> (w379:dbl)
        n209 = local read "左位移零点偏移值"() -> (w375:dbl)
        n210 = Multiply(x=w408, y=1000.0) -> (x*y=w407:dbl)
        n211 = Multiply(x=w415, y=1000.0) -> (x*y=w414:dbl)
        n212 = Subtract(x=w407, y=w376) -> (x-y=w370:dbl)
        n213 = Multiply(x=w384, y=25.0) -> (x*y=w397:dbl)
        n214 = Multiply(x=w386, y=25.0) -> (x*y=w401:dbl)
        n215 = local read "压力1比例偏移值"() -> (w377:dbl)
        n216 = Subtract(x=w414, y=w379) -> (x-y=w371:dbl)
        n217 = local read "右位移比例偏移值"() -> (w372:dbl)
        n218 = Subtract(x=w397, y=w375) -> (x-y=w383:dbl)
        n219 = Subtract(x=w401, y=w373) -> (x-y=w385:dbl)
        n220 = local read "压力2比例偏移值"() -> (w378:dbl)
        n221 = local read "左位移比例偏移值"() -> (w374:dbl)
        n222 = Multiply(x=w370, y=w377) -> (x*y=w366:dbl)
        n223 = Multiply(x=w385, y=w372) -> (x*y=w381:dbl)
        n224 = Multiply(x=w371, y=w378) -> (x*y=w365:dbl)
        n225 = Multiply(x=w383, y=w374) -> (x*y=w380:dbl)
        n226 = Greater Or Equal?(x=w366, y=18.0) -> (x >= y?=→"压力报警2":bool)
        n227 = local write "右实时位移(mm)"(w381) -> ()
        n228 = local write "右实时压力(N)"(w366) -> ()
        n229 = local write "左实时压力(N)"(w365) -> ()
        n230 = local write "左实时位移(mm)"(w380) -> ()
        n231 = Greater Or Equal?(x=w365, y=18.0) -> (x >= y?=→"压力报警1":bool)
        n232 = local read "停止"() -> (w382:bool)
      }
    }
    frame #2 {
      n233 = dll-call lib="PTH17abs DQ14070-Z120人机界面-Z120PCI8622_32.dll" fn="PCI8622_StopDeviceProAD" label="StopDeviceProAD"("hDevice"=w432) -> ("hDevice"=w433:i32)  [unwired: 4 in, 2 out]
      n234 = dll-call lib="PTH17abs DQ14070-Z120人机界面-Z120PCI8622_32.dll" fn="PCI8622_ReleaseDeviceProAD" label="ReleaseDeviceProAD"("hDevice"=w433) -> ()  [unwired: 5 in, 2 out]
    }
    frame #3 {
      n235 = dll-call lib="PTH17abs DQ14070-Z120人机界面-Z120PCI8622_32.dll" fn="PCI8622_ReleaseDevice" label="ReleaseDevice"("hDevice"=w434) -> ()  [unwired: 5 in, 2 out]
    }
  }
  n236 = while {
    stop <- w437 stop-if-true
    n237 = local read "右工步号2700"() -> (w436:u32)
    n238 = case shown="20" w436 {
      frame 0, Default {
      }
      frame 20 {
        n239 = flat-sequence {
          tunnel: [w448] -> w440
          tunnel: [w458] -> w442
          tunnel: [w453] -> w441
          tunnel: w440 -> [w453]
          tunnel: [w462] -> w446
          tunnel: [w461] -> w445
          tunnel: w442 -> [w460]
          tunnel: w441 -> [w459]
          tunnel: w446 -> [w481]
          tunnel: w445 -> [w480]
          tunnel: [w484] -> w444
          tunnel: [w478] -> w438
          tunnel: w444 -> [w496]
          tunnel: [w493] -> w443
          tunnel: [w490] -> w439
          tunnel: w438 -> [w487]
          tunnel: w443 -> [w498]
          tunnel: w439 -> [w497]
          frame #0 {
            w447 = FALSE ("压装合格2")
            n240 = local write "右压装合格"(w447) -> ()
            n241 = local write "右压装不合格"(w447) -> ()
          }
          frame #1 {
            n242 = local read "区域最小压力1(KN)"() -> (w450:dbl)
            n243 = local read "区域最大压力1(KN)"() -> (w449:dbl)
            n244 = local read "区域最小位移1(mm)"() -> (w452:dbl)
            n245 = local read "区域最大位移1(mm)"() -> (w451:dbl)
            n246 = call "区域曲线.vi"("区域最大压力(N)"=w449, "区域最小压力(N)"=w450, "区域最大位移(mm)"=w451, "区域最小位移(mm)"=w452) -> ("区域曲线"=w448:cluster{dbl[], dbl[]})  [unwired: 7 in]
          }
          frame #2 {
            n247 = local read "区域最小压力2(KN)"() -> (w455:dbl)
            n248 = local read "区域最大压力2(KN)"() -> (w454:dbl)
            n249 = local read "区域最小位移2(mm)"() -> (w457:dbl)
            n250 = local read "区域最大位移2(mm)"() -> (w456:dbl)
            n251 = call "区域曲线.vi"("区域最大压力(N)"=w454, "区域最小压力(N)"=w455, "区域最大位移(mm)"=w456, "区域最小位移(mm)"=w457) -> ("区域曲线"=w458:cluster{dbl[], dbl[]})  [unwired: 7 in]
          }
          frame #3 {
            w463 = dbl[] []
            n252 = while {
              shift-right: [w475] -> w462
              shift-left: w463 -> [w476]
              shift-right: [w473] -> w461
              shift-left: w463 -> [w474]
              tunnel: w460 -> [w465]
              tunnel: w459 -> [w464]
              stop <- w470 stop-if-true
              n253 = local read "右实时压力(N)"() -> (w468:dbl)
              n254 = local read "右实时位移(mm)"() -> (w467:dbl)
              n255 = local read "右工步号2700"() -> (w472:u32)
              n256 = Build Array (concatenate)(w476, w467) -> (w475:dbl[])
              n257 = Build Array (concatenate)(w474, w468) -> (w473:dbl[])
              n258 = Equal?(x=w472, y=30.0) -> (x = y?=w470:bool)
              n259 = Bundle(w475, w473) -> (w477:cluster{dbl[], dbl[]})  [unwired: 1 in]
              n260 = Build Array(w477, w465, w464) -> (→"右压力位移曲线":cluster{dbl[], dbl[]}[])
              n261 = Wait Until Next ms Multiple(millisecond multiple=u32 50 ("毫秒倍数")) -> ()  [unwired: 1 out]
            }
          }
          frame #4 {
            n262 = local read "位移监控点2(mm)"() -> (w483:dbl)
            n263 = local read "位移监控点1(mm)"() -> (w479:dbl)
            n264 = Array Max & Min "数组最大值与最小值"(array=w481) -> (max value=→"右实测压入位移(mm)":dbl)  [unwired: 3 out]
            n265 = call "压力位移插值.vi"("压力数组"=w480, "监控点位移"=w479, "位移数组"=w481) -> ("监控点压力"=w478:dbl)  [unwired: 2 in]
            "右实测监控点压力1(KN)" <- w478
            n266 = call "压力位移插值.vi"("压力数组"=w480, "监控点位移"=w483, "位移数组"=w481) -> ("监控点压力"=w484:dbl)  [unwired: 2 in]
            "右实测监控点压力2(KN)" <- w484
            "右位移参数组" <- w481
            "右压力参数组" <- w480
          }
          frame #5 {
            n267 = local read "监控点最小压力2(KN)"() -> (w486:dbl)
            n268 = local read "监控点最大压力2(KN)"() -> (w485:dbl)
            n269 = local read "监控点最小压力1(KN)"() -> (w489:dbl)
            n270 = local read "监控点最大压力1(KN)"() -> (w488:dbl)
            n271 = Less Or Equal?(x=w486, y=w496) -> (x <= y?=w495:bool)
            n272 = Less Or Equal?(x=w496, y=w485) -> (x <= y?=w494:bool)
            n273 = Less Or Equal?(x=w489, y=w487) -> (x <= y?=w491:bool)
            n274 = Less Or Equal?(x=w487, y=w488) -> (x <= y?=w492:bool)
            n275 = And(x=w495, y=w494) -> (x .and. y?=w493:bool)
            n276 = And(x=w491, y=w492) -> (x .and. y?=w490:bool)
          }
          frame #6 {
            n277 = And(x=w498, y=w497) -> (x .and. y?=w499:bool)
            "右压装合格" <- w499
            n278 = Not(x=w499) -> (.not. x?=→"右压装不合格":bool)
          }
          frame #7 {
            n279 = local write "右工步号2700"(40.0 ("工步2序号")) -> ()
          }
        }
      }
    }
    n280 = local read "停止"() -> (w437:bool)
    n281 = Wait Until Next ms Multiple(millisecond multiple=u32 50 ("毫秒倍数")) -> ()  [unwired: 1 out]
  }
  n282 = while {
    stop <- w502 stop-if-true
    n283 = local read "自动工步号"() -> (w503:u32)
    n284 = local read "停止"() -> (w502:bool)
    n285 = case shown="105" w503 {
      frame 0, Default {
      }
      frame 40 {
        n286 = Get Date/Time In Seconds() -> (seconds since 1Jan1904=w506:timestamp)
        n287 = Format Date/Time String(time format string (%c)="%Y%m%d%H%M" ("时间格式字符串(%c)"), seconds (now)=w506) -> (date/time string=w504:string)  [unwired: 1 in]
        n288 = local write "KSSJ"(w504) -> ()
      }
      frame 105 {
        n289 = flat-sequence {
          tunnel: [w524] -> w521
          tunnel: [w522] -> w520
          tunnel: w521 -> [w530]
          tunnel: w520 -> [w529]
          tunnel: [w530] -> w519
          tunnel: [w529] -> w518
          tunnel: ["F:\\报表存储\\" ("字符串")] -> w517
          tunnel: w519 -> [w543]
          tunnel: w518 -> [w537]
          tunnel: w517 -> [w542]
          tunnel: [w541] -> w516
          tunnel: [w539] -> w515
          tunnel: [w535] -> w514
          tunnel: [w531] -> w513
          tunnel: w516 -> [w549]
          tunnel: [w550] -> w512
          tunnel: w515 -> [w550]
          tunnel: w514 -> [w548]
          tunnel: [w547] -> w511
          tunnel: w513 -> [w546]
          tunnel: [w545] -> w510
          tunnel: [w564] -> w509
          tunnel: w512 -> [w564]
          tunnel: w511 -> [w563]
          tunnel: [w563] -> w508
          tunnel: [w562] -> w507
          tunnel: w510 -> [w562]
          tunnel: w509 -> [w571]
          tunnel: w508 -> [w570]
          tunnel: w507 -> [w567]
          frame #0 {
            n290 = local read "产品ID"() -> (w523:string)
            n291 = Format Date/Time String(time format string (%c)="%Y%m%d" ("时间格式字符串(%c)")) -> (date/time string=w525:string)  [unwired: 2 in]
            n292 = call <vilib>:"Trim Whitespace.vi"("string"=w523) -> ("trimmed string"=w522:string)  [unwired: 1 in]
            n293 = String Subset(string=w525, offset (0)=0 ("偏移量(0)")) -> (substring=w524:string)  [unwired: 1 in]
          }
          frame #1 {
          }
          frame #2 {
            w538 = "\\" ("字符串")
            n294 = Concatenate Strings(w542, w543, w538, w537, w538) -> (w532:string)
            n295 = Concatenate Strings(w542, w543, w538, w537, w538) -> (w544:string)
            n296 = String To Path(string=w544) -> (path=w541:path)
            n297 = Concatenate Strings(w532, "压力位移曲线.DOC" ("字符串")) -> (w540:string)
            n298 = Concatenate Strings(w532, "右压力位移数组.txt" ("字符串")) -> (w531:string)
            n299 = Concatenate Strings(w532, "左压力位移数组.txt" ("字符串")) -> (w535:string)
            n300 = String To Path(string=w540) -> (path=w539:path)
          }
          frame #3 {
            n301 = call <vilib>:"Check if File or Folder Exists.vi"("path"=w549) -> ("file or folder exists?"=w551:bool)  [unwired: 8 in, 2 out]
            n302 = String To Path(string=w548) -> (path=w547:path)
            n303 = String To Path(string=w546) -> (path=w545:path)
            n304 = case shown="真" w551 {
              tunnel: w549 -> [w552 w553]
              frame False {
                n305 = Create Folder(path (use dialog)=w552) -> ()  [unwired: 2 in, 3 out]
              }
              frame True {
                n306 = flat-sequence {
                  tunnel: w553 -> [w557]
                  tunnel: [w555] -> w554
                  tunnel: w554 -> [w560]
                  frame #0 {
                    n307 = Delete(path (use dialog)=w557, entire hierarchy (F)=TRUE ("整个层次结构(F)")) -> (deleted path=w555:path)  [unwired: 3 in, 2 out]
                  }
                  frame #1 {
                    n308 = call <vilib>:"Check if File or Folder Exists.vi"("path"=w560) -> ("file or folder exists?"=w559:bool, "dup path"=w558:path)  [unwired: 8 in, 1 out]
                    n309 = case shown="假" w559 {
                      tunnel: w558 -> [w561 _]
                      frame False {
                        n310 = Create Folder(path (use dialog)=w561) -> ()  [unwired: 2 in, 3 out]
                      }
                      frame True {
                      }
                    }
                  }
                }
              }
            }
          }
          frame #4 {
            n311 = Wait Until Next ms Multiple(millisecond multiple=u32 1000 ("毫秒倍数")) -> ()  [unwired: 1 out]
          }
          frame #5 {
            n312 = flat-sequence {
              tunnel: w570 -> [w574]
              tunnel: w571 -> [w575]
              tunnel: [w575] -> w569
              tunnel: [w574] -> w568
              tunnel: w567 -> [w572]
              tunnel: [w572] -> w566
              tunnel: w569 -> [w582]
              tunnel: w568 -> [w576]
              tunnel: w566 -> [w579]
              frame #0 {
                n313 = local write "选项卡控件"(T1."自动界面" ("选项卡控件")) -> ()
              }
              frame #1 {
                w585 = T3 2 items=["快速打印", "标准报表", "HTML", "双字节", "Excel"] ("report type (Quick Print)")
                w584 = T4 1 items=["完整前面板", "前面板可见部分", "图标、说明、前面板和程序框图", "说明信息: 使用前面板", "说明信息: 作为子VI使用", "说明信息: 完整", "说明信息: 自定义"] ("contents (complete front panel)")
                n314 = local read "左位移参数组"() -> (w580:dbl[])
                n315 = local read "左压力参数组"() -> (w581:dbl[])
                n316 = local read "右位移参数组"() -> (w577:dbl[])
                n317 = local read "右压力参数组"() -> (w578:dbl[])
                n318 = call "导出曲线数组.vi"("压力参数"=w581, "位移参数"=w580, "file path (dialog if empty)"=w576) -> ()  [unwired: 17 in]
                n319 = call "导出曲线数组.vi"("压力参数"=w578, "位移参数"=w577, "file path (dialog if empty)"=w579) -> ()  [unwired: 17 in]
                n320 = Current VI's Path() -> (path=w583:path)
                n321 = call-poly <vilib>:"Easy Print VI Panel or Documentation.vi"("report type (Quick Print)"=w585, "contents (complete front panel)"=w584, "VI path"=w583) -> ("error out"=w587:errorcluster, "report out"=w586:refnum<class "NI_report.lvclass">)  [unwired: 1 in, 6 out]
                n322 = call-dynamic "Save Report to File.vi"("report in"=w586, "report file path"=w582, "error in (no error)"=w587) -> ()  [unwired: 2 in, 11 out]
              }
            }
          }
          frame #6 {
            n323 = local write "自动工步号"(110.0 ("工步号")) -> ()
          }
        }
      }
      frame 116 {
        n324 = flat-sequence {
          tunnel: [w612] -> w589
          tunnel: w589 -> [w621]
          frame #0 {
            n325 = local read "左压装合格"() -> (w592:bool)
            n326 = local read "右压装合格"() -> (w591:bool)
            n327 = Compound Arithmetic op=AND(w592, w591) -> (w590:bool)
            n328 = local write "本序合格"(w590) -> ()
          }
          frame #1 {
            n329 = while {
              stop <- w594 stop-if-true
              n330 = Get Date/Time In Seconds() -> (seconds since 1Jan1904=w599:timestamp)
              n331 = local read "JSSJ"() -> (w596:string)
              n332 = Format Date/Time String(time format string (%c)="%Y%m%d%H%M" ("时间格式字符串(%c)"), seconds (now)=w599) -> (date/time string=w597:string)  [unwired: 1 in]
              n333 = Wait Until Next ms Multiple(millisecond multiple=u32 50 ("毫秒倍数")) -> ()  [unwired: 1 out]
              n334 = Not Equal?(x=w596, y="") -> (x != y?=w594:bool)
              n335 = local write "JSSJ"(w597) -> ()
            }
          }
          frame #2 {
            w608 = i16 4 ("精度(6)")
            n336 = local read "左实测监控点压力1(KN)"() -> (w607:dbl)
            n337 = local read "左实测监控点压力2(KN)"() -> (w602:dbl)
            n338 = local read "右实测监控点压力1(KN)"() -> (w601:dbl)
            n339 = local read "右实测监控点压力2(KN)"() -> (w600:dbl)
            n340 = local read "本序合格"() -> (w616:bool)
            n341 = local read "员工ID"() -> (w617:string)
            n342 = local read "产品ID"() -> (w618:string)
            n343 = local read "KSSJ"() -> (w615:string)
            n344 = local read "JSSJ"() -> (w610:string)
            n345 = local read "FGCS"() -> (w614:string)
            n346 = Boolean To (0,1)(Boolean=w616) -> (0, 1=w620:i16)
            n347 = Number To Decimal String(number=w620, width (-)=i16 1 ("宽度(-)")) -> (decimal integer string=w609:string)
            n348 = Number To Fractional String(number=w607, precision (6)=w608) -> (F-format string=w606:string)  [unwired: 2 in]
            n349 = Number To Fractional String(number=w602, precision (6)=w608) -> (F-format string=w605:string)  [unwired: 2 in]
            n350 = Number To Fractional String(number=w601, precision (6)=w608) -> (F-format string=w604:string)  [unwired: 2 in]
            n351 = Number To Fractional String(number=w600, precision (6)=w608) -> (F-format string=w603:string)  [unwired: 2 in]
            n352 = Build Array(w618, w617, w609, "1", w615, w610, w614, "Q14073-12", w606, w605, w604, w603) -> (w612:string[])
          }
          frame #3 {
            n353 = Wait (ms)(milliseconds to wait=u32 500 ("等待时间（毫秒）")) -> ()  [unwired: 1 out]
            n354 = call "数据库更新.vi"("设备号"="10", "数据"=w621) -> ()  [unwired: 13 in, 1 out]
          }
          frame #4 {
            n355 = local write "自动工步号"(120.0 ("工步号")) -> ()
          }
        }
      }
    }
  }
